vi "Motors Find Datums.vi"(1 "Creep Speed 4":dbl, 2 "Creep Speed 3":dbl, 4 "error in":errorcluster, 5 "Creep Speed 2":dbl, 6 "Creep Speed":dbl, 7 "VISA in":refnum<visa-resource-name>) -> (0 "error out":errorcluster, 3 "VISA out":refnum<visa-resource-name>)   [LabVIEW 2018]
panel:
  out "read buffer":string
  in  "Wait time Theta (s)":i32=1200
  in  "Wait time X (s)":i32=1200
  in  "Wait time Z (s)":i32=1200
  in  "Wait time Y (s)":i32=1200
  out "SV 4":string
  out "DM 4":string
  out "HD 4":string
  out "SV 2":string
  out "HD 1":string
  out "SV 3":string
  out "DM 3":string
  out "HD 3":string
  out "DM 1":string
  out "SV 1":string
  out "HD 2":string
  out "DM 2":string
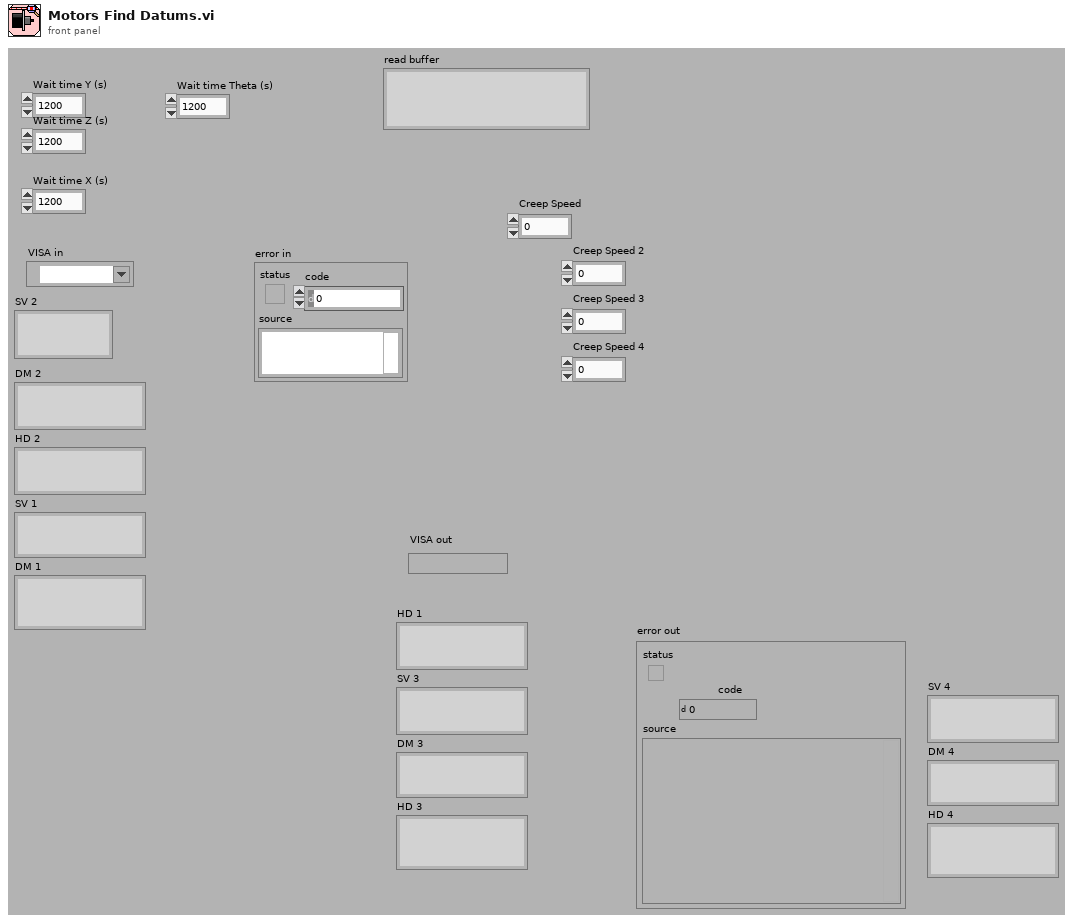
[diagram p1: front panel]
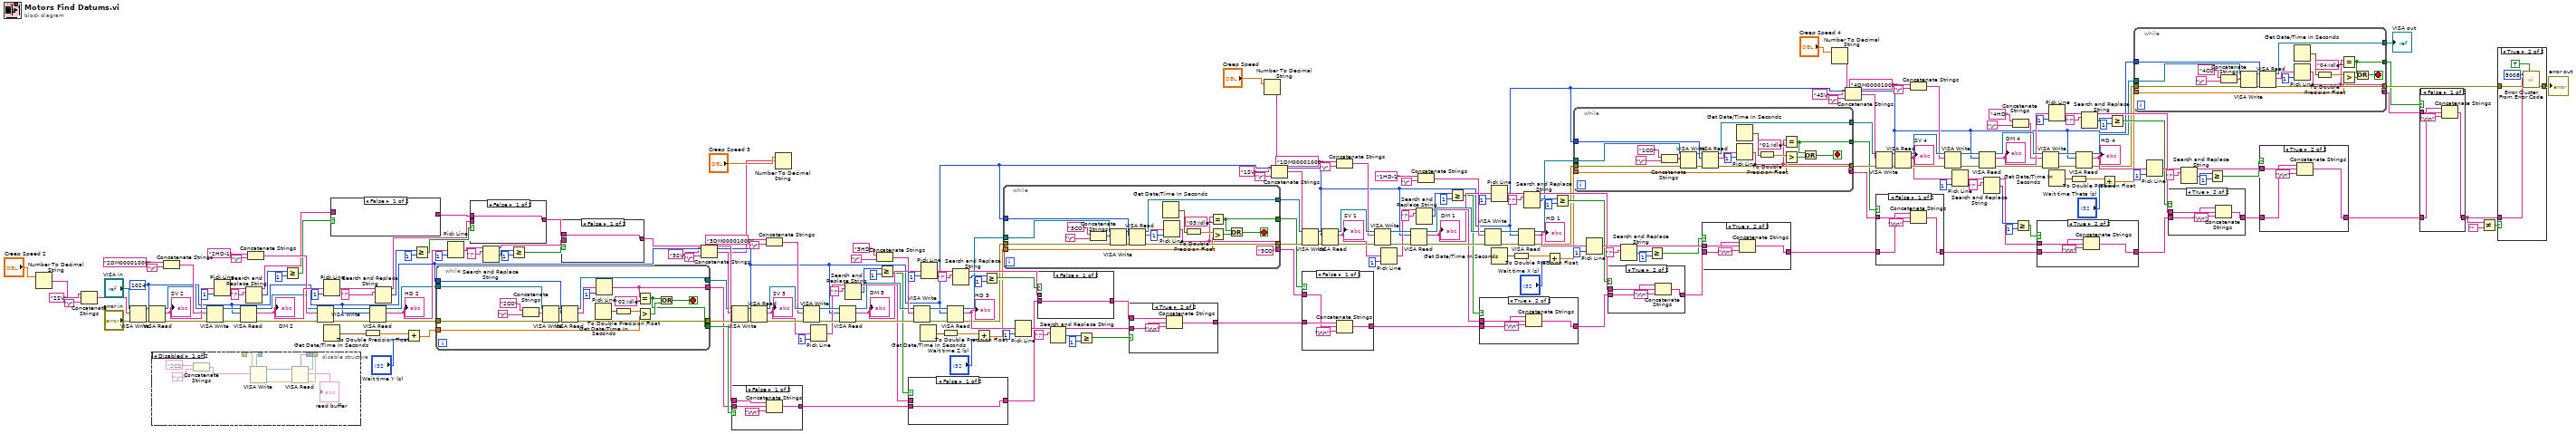
[diagram p0: block diagram]
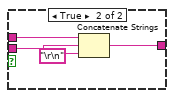
[diagram p8: hidden frame]
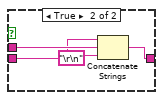
[diagram p13: hidden frame]
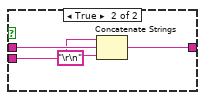
[diagram p14: hidden frame]
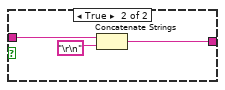
[diagram p18: hidden frame]
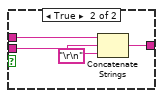
[diagram p19: hidden frame]
diagram:
  w15 = u32 1024 ("byte count")
  n1 = Number To Decimal String(number="Creep Speed 2") -> (decimal integer string=w10:string)  [unwired: 1 in]
  n2 = Concatenate Strings("2SV" ("write buffer"), w10, "\r") -> (w180:string)
  n3 = VISA Write(VISA resource name="VISA in", write buffer=w180, error in (no error)="error in") -> (VISA resource name out=w193:refnum<visa-resource-name>, error out=w192:errorcluster)  [unwired: 1 out]
  n4 = VISA Read(VISA resource name=w193, byte count=w15, error in (no error)=w192) -> (VISA resource name out=w190:refnum<visa-resource-name>, read buffer=w181:string, error out=w188:errorcluster)  [unwired: 1 out]
  "SV 2" <- w181
  n5 = disable-structure shown="Disabled" {
    disable-tunnel: _ -> [w251 _]
    disable-tunnel: _ -> [w250 _]
    disable-tunnel: _ -> [w249 _]
    disable-tunnel: [w248 _] -> _
    disable-tunnel: [w247 _] -> _
    frame Disabled {
      n6 = Concatenate Strings("2CD" ("string"), "\r") -> (w245:string)
      n7 = VISA Write(VISA resource name=w250, write buffer=w245, error in (no error)=w249) -> (VISA resource name out=w253:refnum<visa-resource-name>, error out=w252:errorcluster)  [unwired: 1 out]
      n8 = VISA Read(VISA resource name=w253, byte count=w251, error in (no error)=w252) -> (VISA resource name out=w248:refnum<visa-resource-name>, read buffer=→"read buffer":string, error out=w247:errorcluster)  [unwired: 1 out]
    }
    frame Enabled {
    }
  }
  n9 = Concatenate Strings("2DM00001000" ("Initial command 1"), "\r") -> (w204:string)
  n10 = VISA Write(VISA resource name=w190, write buffer=w204, error in (no error)=w188) -> (VISA resource name out=w239:refnum<visa-resource-name>, error out=w240:errorcluster)  [unwired: 1 out]
  n11 = Pick Line(multi-line string=w181, line index=1) -> (output string=w183:string)  [unwired: 1 in]
  n12 = VISA Read(VISA resource name=w239, byte count=w15, error in (no error)=w240) -> (VISA resource name out=w14:refnum<visa-resource-name>, read buffer=w203:string, error out=w13:errorcluster)  [unwired: 1 out]
  "DM 2" <- w203
  n13 = Search and Replace String(input string=w183, search string="!") -> (result string=w185:string, number of replacements=w186:i32)  [unwired: 6 in, 2 out]
  n14 = Concatenate Strings("2HD-1" ("Initial command 1"), "\r") -> (w194:string)
  n15 = Greater Or Equal?(x=w186, y=1) -> (x >= y?=w68:bool)
  n16 = VISA Write(VISA resource name=w14, write buffer=w194, error in (no error)=w13) -> (VISA resource name out=w238:refnum<visa-resource-name>, error out=w237:errorcluster)  [unwired: 1 out]
  n17 = Get Date/Time In Seconds() -> (seconds since 1Jan1904=w63:timestamp)
  n18 = Pick Line(multi-line string=w203, line index=1) -> (output string=w201:string)  [unwired: 1 in]
  n19 = case shown="False" w68 {
    tunnel: w185 -> [_ w255]
    tunnel: [_ w254] -> w86
    frame False {
    }
    frame True {
      n20 = Concatenate Strings(w255, "\r\n") -> (w254:string)
    }
  }
  n21 = To Double Precision Float(number=w63) -> (double precision float=w62:dbl)
  n22 = VISA Read(VISA resource name=w238, byte count=w15, error in (no error)=w237) -> (VISA resource name out=w64:refnum<visa-resource-name>, read buffer=w87:string, error out=w65:errorcluster)  [unwired: 1 out]
  "HD 2" <- w87
  n23 = Search and Replace String(input string=w201, search string="!") -> (result string=w199:string, number of replacements=w198:i32)  [unwired: 6 in, 2 out]
  n24 = Add(x=w62, y="Wait time Y (s)") -> (x+y=w61:dbl)
  n25 = Greater Or Equal?(x=w198, y=1) -> (x >= y?=w69:bool)
  n26 = while {
    tunnel: w65 -> [w276]
    tunnel: w64 -> [w275]
    tunnel: w15 -> [w261]
    tunnel: [w262] -> w57
    tunnel: [w263] -> w56
    tunnel: w61 -> [w272]
    tunnel: [w268] -> w37
    tunnel: [w266] -> w36
    stop <- w269 stop-if-true
    n27 = Concatenate Strings("2CO" ("write buffer"), "\r") -> (w258:string)
    n28 = VISA Write(VISA resource name=w275, write buffer=w258, error in (no error)=w276) -> (VISA resource name out=w265:refnum<visa-resource-name>, error out=w264:errorcluster)  [unwired: 1 out]
    n29 = VISA Read(VISA resource name=w265, byte count=w261, error in (no error)=w264) -> (VISA resource name out=w262:refnum<visa-resource-name>, read buffer=w260:string, error out=w263:errorcluster)  [unwired: 1 out]
    n30 = Get Date/Time In Seconds() -> (seconds since 1Jan1904=w273:timestamp)
    n31 = Pick Line(multi-line string=w260, line index=1) -> (output string=w266:string)  [unwired: 1 in]
    n32 = To Double Precision Float(number=w273) -> (double precision float=w271:dbl)
    n33 = Equal?(x=w266, y="02:Idle") -> (x = y?=w268:bool)
    n34 = Greater?(x=w271, y=w272) -> (0:w270:bool)
    n35 = Or(x=w268, y=w270) -> (x .or. y?=w269:bool)
  }
  n36 = Pick Line(multi-line string=w87, line index=1) -> (output string=w93:string)  [unwired: 1 in]
  n37 = case shown="False" w69 {
    tunnel: w199 -> [_ w280]
    tunnel: w86 -> [w277 w281]
    tunnel: [w277 w278] -> w85
    frame False {
    }
    frame True {
      n38 = Concatenate Strings(w281, w280, "\r\n") -> (w278:string)
    }
  }
  n39 = Search and Replace String(input string=w93, search string="!") -> (result string=w91:string, number of replacements=w90:i32)  [unwired: 6 in, 2 out]
  n40 = Greater Or Equal?(x=w90, y=1) -> (x >= y?=w67:bool)
  n41 = case shown="False" w67 {
    tunnel: w91 -> [_ w284]
    tunnel: w85 -> [w282 w285]
    tunnel: [w282 w283] -> w35
    frame False {
    }
    frame True {
      n42 = Concatenate Strings(w285, w284, "\r\n") -> (w283:string)
    }
  }
  n43 = case shown="False" w37 {
    tunnel: w36 -> [w288 _]
    tunnel: w35 -> [w289 w291]
    tunnel: [w287 w291] -> w30
    frame False {
      n44 = Concatenate Strings(w289, w288, "\r\n") -> (w287:string)
    }
    frame True {
    }
  }
  n45 = Concatenate Strings("3DM00001000" ("Initial command 3"), "\r") -> (w219:string)
  n46 = Number To Decimal String(number="Creep Speed 3") -> (decimal integer string=w7:string)  [unwired: 1 in]
  n47 = Concatenate Strings("3SV" ("Initial command 2"), w7, "\r") -> (w216:string)
  n48 = VISA Write(VISA resource name=w57, write buffer=w216, error in (no error)=w56) -> (VISA resource name out=w213:refnum<visa-resource-name>, error out=w214:errorcluster)  [unwired: 1 out]
  n49 = VISA Read(VISA resource name=w213, byte count=w15, error in (no error)=w214) -> (VISA resource name out=w221:refnum<visa-resource-name>, read buffer=w147:string, error out=w220:errorcluster)  [unwired: 1 out]
  "SV 3" <- w147
  n50 = VISA Write(VISA resource name=w221, write buffer=w219, error in (no error)=w220) -> (VISA resource name out=w223:refnum<visa-resource-name>, error out=w222:errorcluster)  [unwired: 1 out]
  n51 = Pick Line(multi-line string=w147, line index=1) -> (output string=w152:string)  [unwired: 1 in]
  n52 = VISA Read(VISA resource name=w223, byte count=w15, error in (no error)=w222) -> (VISA resource name out=w224:refnum<visa-resource-name>, read buffer=w140:string, error out=w225:errorcluster)  [unwired: 1 out]
  "DM 3" <- w140
  n53 = Search and Replace String(input string=w152, search string="!") -> (result string=w150:string, number of replacements=w149:i32)  [unwired: 6 in, 2 out]
  n54 = Concatenate Strings("3HD" ("Initial command 4"), "\r") -> (w229:string)
  n55 = Greater Or Equal?(x=w149, y=1) -> (x >= y?=w73:bool)
  n56 = case shown="False" w73 {
    tunnel: w150 -> [_ w295]
    tunnel: [w292 w294] -> w82
    tunnel: w30 -> [w292 w293]
    frame False {
    }
    frame True {
      n57 = Concatenate Strings(w293, w295, "\r\n") -> (w294:string)
    }
  }
  n58 = VISA Write(VISA resource name=w224, write buffer=w229, error in (no error)=w225) -> (VISA resource name out=w227:refnum<visa-resource-name>, error out=w226:errorcluster)  [unwired: 1 out]
  n59 = Get Date/Time In Seconds() -> (seconds since 1Jan1904=w58:timestamp)
  n60 = Pick Line(multi-line string=w140, line index=1) -> (output string=w142:string)  [unwired: 1 in]
  n61 = To Double Precision Float(number=w58) -> (double precision float=w59:dbl)
  n62 = VISA Read(VISA resource name=w227, byte count=w15, error in (no error)=w226) -> (VISA resource name out=w55:refnum<visa-resource-name>, read buffer=w133:string, error out=w54:errorcluster)  [unwired: 1 out]
  "HD 3" <- w133
  n63 = Search and Replace String(input string=w142, search string="!") -> (result string=w144:string, number of replacements=w145:i32)  [unwired: 6 in, 2 out]
  n64 = Add(x=w59, y="Wait time Z (s)") -> (x+y=w60:dbl)
  n65 = Greater Or Equal?(x=w145, y=1) -> (x >= y?=w74:bool)
  n66 = while {
    tunnel: w54 -> [w316]
    tunnel: w55 -> [w303]
    tunnel: w15 -> [w315]
    tunnel: [w309] -> w53
    tunnel: [w308] -> w52
    tunnel: w60 -> [w306]
    tunnel: [w301] -> w34
    tunnel: [w300] -> w33
    stop <- w304 stop-if-true
    (unwired) "3CO" ("write buffer")
    n67 = Concatenate Strings("3CO" ("write buffer"), "\r") -> (w297:string)
    n68 = VISA Write(VISA resource name=w303, write buffer=w297, error in (no error)=w316) -> (VISA resource name out=w314:refnum<visa-resource-name>, error out=w313:errorcluster)  [unwired: 1 out]
    n69 = VISA Read(VISA resource name=w314, byte count=w315, error in (no error)=w313) -> (VISA resource name out=w309:refnum<visa-resource-name>, read buffer=w311:string, error out=w308:errorcluster)  [unwired: 1 out]
    n70 = Get Date/Time In Seconds() -> (seconds since 1Jan1904=w307:timestamp)
    n71 = Pick Line(multi-line string=w311, line index=1) -> (output string=w300:string)  [unwired: 1 in]
    n72 = To Double Precision Float(number=w307) -> (double precision float=w302:dbl)
    n73 = Equal?(x=w300, y="03:Idle") -> (x = y?=w301:bool)
    n74 = Greater?(x=w302, y=w306) -> (0:w305:bool)
    n75 = Or(x=w301, y=w305) -> (x .or. y?=w304:bool)
  }
  n76 = Pick Line(multi-line string=w133, line index=1) -> (output string=w138:string)  [unwired: 1 in]
  n77 = case shown="False" w74 {
    tunnel: w144 -> [_ w320]
    tunnel: [w317 w319] -> w81
    tunnel: w82 -> [w317 w318]
    frame False {
    }
    frame True {
      n78 = Concatenate Strings(w318, w320, "\r\n") -> (w319:string)
    }
  }
  n79 = Search and Replace String(input string=w138, search string="!") -> (result string=w136:string, number of replacements=w135:i32)  [unwired: 6 in, 2 out]
  n80 = Greater Or Equal?(x=w135, y=1) -> (x >= y?=w75:bool)
  n81 = case shown="True" w75 {
    tunnel: w136 -> [_ w325]
    tunnel: w81 -> [w322 w324]
    tunnel: [w322 w323] -> w32
    frame False {
    }
    frame True {
      n82 = Concatenate Strings(w324, w325, "\r\n") -> (w323:string)
    }
  }
  n83 = Number To Decimal String(number="Creep Speed") -> (decimal integer string=w4:string)  [unwired: 1 in]
  n84 = Concatenate Strings("1SV" ("write buffer"), w4, "\r") -> (w177:string)
  n85 = VISA Write(VISA resource name=w53, write buffer=w177, error in (no error)=w52) -> (VISA resource name out=w235:refnum<visa-resource-name>, error out=w236:errorcluster)  [unwired: 1 out]
  n86 = case shown="False" w34 {
    tunnel: w33 -> [w328 _]
    tunnel: w32 -> [w329 w331]
    tunnel: [w327 w331] -> w31
    frame False {
      n87 = Concatenate Strings(w329, w328, "\r\n") -> (w327:string)
    }
    frame True {
    }
  }
  n88 = VISA Read(VISA resource name=w235, byte count=w15, error in (no error)=w236) -> (VISA resource name out=w234:refnum<visa-resource-name>, read buffer=w170:string, error out=w233:errorcluster)  [unwired: 1 out]
  "SV 1" <- w170
  n89 = Concatenate Strings("1DM00001000" ("Initial command 1"), "\r") -> (w169:string)
  n90 = VISA Write(VISA resource name=w234, write buffer=w169, error in (no error)=w233) -> (VISA resource name out=w231:refnum<visa-resource-name>, error out=w232:errorcluster)  [unwired: 1 out]
  n91 = Pick Line(multi-line string=w170, line index=1) -> (output string=w172:string)  [unwired: 1 in]
  n92 = VISA Read(VISA resource name=w231, byte count=w15, error in (no error)=w232) -> (VISA resource name out=w208:refnum<visa-resource-name>, read buffer=w162:string, error out=w207:errorcluster)  [unwired: 1 out]
  "DM 1" <- w162
  n93 = Search and Replace String(input string=w172, search string="!") -> (result string=w174:string, number of replacements=w175:i32)  [unwired: 6 in, 2 out]
  n94 = Concatenate Strings("1HD-1" ("Initial command 1"), "\r") -> (w210:string)
  n95 = Greater Or Equal?(x=w175, y=1) -> (x >= y?=w70:bool)
  n96 = case shown="True" w70 {
    tunnel: w174 -> [_ w335]
    tunnel: [w332 w334] -> w84
    tunnel: w31 -> [w332 w333]
    frame False {
    }
    frame True {
      n97 = Concatenate Strings(w333, w335, "\r\n") -> (w334:string)
    }
  }
  n98 = VISA Write(VISA resource name=w208, write buffer=w210, error in (no error)=w207) -> (VISA resource name out=w212:refnum<visa-resource-name>, error out=w211:errorcluster)  [unwired: 1 out]
  n99 = Get Date/Time In Seconds() -> (seconds since 1Jan1904=w51:timestamp)
  n100 = Pick Line(multi-line string=w162, line index=1) -> (output string=w167:string)  [unwired: 1 in]
  n101 = To Double Precision Float(number=w51) -> (double precision float=w50:dbl)
  n102 = VISA Read(VISA resource name=w212, byte count=w15, error in (no error)=w211) -> (VISA resource name out=w48:refnum<visa-resource-name>, read buffer=w154:string, error out=w47:errorcluster)  [unwired: 1 out]
  "HD 1" <- w154
  n103 = Search and Replace String(input string=w167, search string="!") -> (result string=w165:string, number of replacements=w164:i32)  [unwired: 6 in, 2 out]
  n104 = Add(x=w50, y="Wait time X (s)") -> (x+y=w49:dbl)
  n105 = Greater Or Equal?(x=w164, y=1) -> (x >= y?=w71:bool)
  n106 = while {
    tunnel: w47 -> [w356]
    tunnel: w48 -> [w342]
    tunnel: w15 -> [w355]
    tunnel: [w349] -> w46
    tunnel: [w348] -> w45
    tunnel: w49 -> [w346]
    tunnel: [w341] -> w29
    tunnel: [w340] -> w27
    stop <- w343 stop-if-true
    n107 = Concatenate Strings("1CO" ("write buffer"), "\r") -> (w337:string)
    n108 = VISA Write(VISA resource name=w342, write buffer=w337, error in (no error)=w356) -> (VISA resource name out=w354:refnum<visa-resource-name>, error out=w353:errorcluster)  [unwired: 1 out]
    n109 = VISA Read(VISA resource name=w354, byte count=w355, error in (no error)=w353) -> (VISA resource name out=w349:refnum<visa-resource-name>, read buffer=w351:string, error out=w348:errorcluster)  [unwired: 1 out]
    n110 = Get Date/Time In Seconds() -> (seconds since 1Jan1904=w347:timestamp)
    n111 = Pick Line(multi-line string=w351, line index=1) -> (output string=w341:string)  [unwired: 1 in]
    n112 = To Double Precision Float(number=w347) -> (double precision float=w345:dbl)
    n113 = Equal?(x=w341, y="01:Idle") -> (x = y?=w340:bool)
    n114 = Greater?(x=w345, y=w346) -> (0:w344:bool)
    n115 = Or(x=w340, y=w344) -> (x .or. y?=w343:bool)
  }
  n116 = Pick Line(multi-line string=w154, line index=1) -> (output string=w156:string)  [unwired: 1 in]
  n117 = case shown="True" w71 {
    tunnel: w165 -> [_ w360]
    tunnel: [w357 w359] -> w83
    tunnel: w84 -> [w357 w358]
    frame False {
    }
    frame True {
      n118 = Concatenate Strings(w358, w360, "\r\n") -> (w359:string)
    }
  }
  n119 = Search and Replace String(input string=w156, search string="!") -> (result string=w158:string, number of replacements=w159:i32)  [unwired: 6 in, 2 out]
  n120 = Greater Or Equal?(x=w159, y=1) -> (x >= y?=w72:bool)
  n121 = case shown="True" w72 {
    tunnel: w158 -> [_ w365]
    tunnel: [w362 w364] -> w28
    tunnel: w83 -> [w362 w363]
    frame False {
    }
    frame True {
      n122 = Concatenate Strings(w363, w365, "\r\n") -> (w364:string)
    }
  }
  n123 = Number To Decimal String(number="Creep Speed 4") -> (decimal integer string=w1:string)  [unwired: 1 in]
  n124 = Concatenate Strings("4SV" ("Initial command 2"), w1, "\r") -> (w121:string)
  n125 = VISA Write(VISA resource name=w46, write buffer=w121, error in (no error)=w45) -> (VISA resource name out=w132:refnum<visa-resource-name>, error out=w131:errorcluster)  [unwired: 1 out]
  n126 = case shown="False" w27 {
    tunnel: w29 -> [w368 _]
    tunnel: w28 -> [w369 w371]
    tunnel: [w367 w371] -> w26
    frame False {
      n127 = Concatenate Strings(w369, w368, "\r\n") -> (w367:string)
    }
    frame True {
    }
  }
  n128 = VISA Read(VISA resource name=w132, byte count=w15, error in (no error)=w131) -> (VISA resource name out=w129:refnum<visa-resource-name>, read buffer=w114:string, error out=w130:errorcluster)  [unwired: 1 out]
  "SV 4" <- w114
  n129 = Concatenate Strings("4DM00001000" ("Initial command 3"), "\r") -> (w111:string)
  n130 = VISA Write(VISA resource name=w129, write buffer=w111, error in (no error)=w130) -> (VISA resource name out=w127:refnum<visa-resource-name>, error out=w128:errorcluster)  [unwired: 1 out]
  n131 = Pick Line(multi-line string=w114, line index=1) -> (output string=w116:string)  [unwired: 1 in]
  n132 = VISA Read(VISA resource name=w127, byte count=w15, error in (no error)=w128) -> (VISA resource name out=w126:refnum<visa-resource-name>, read buffer=w104:string, error out=w125:errorcluster)  [unwired: 1 out]
  "DM 4" <- w104
  n133 = Search and Replace String(input string=w116, search string="!") -> (result string=w118:string, number of replacements=w119:i32)  [unwired: 6 in, 2 out]
  n134 = Concatenate Strings("4HD" ("Initial command 4"), "\r") -> (w101:string)
  n135 = Greater Or Equal?(x=w119, y=1) -> (x >= y?=w76:bool)
  n136 = case shown="True" w76 {
    tunnel: w118 -> [_ w375]
    tunnel: [w372 w374] -> w80
    tunnel: w26 -> [w372 w373]
    frame False {
    }
    frame True {
      n137 = Concatenate Strings(w373, w375, "\r\n") -> (w374:string)
    }
  }
  n138 = VISA Write(VISA resource name=w126, write buffer=w101, error in (no error)=w125) -> (VISA resource name out=w123:refnum<visa-resource-name>, error out=w124:errorcluster)  [unwired: 1 out]
  n139 = Get Date/Time In Seconds() -> (seconds since 1Jan1904=w42:timestamp)
  n140 = Pick Line(multi-line string=w104, line index=1) -> (output string=w109:string)  [unwired: 1 in]
  n141 = To Double Precision Float(number=w42) -> (double precision float=w43:dbl)
  n142 = VISA Read(VISA resource name=w123, byte count=w15, error in (no error)=w124) -> (VISA resource name out=w41:refnum<visa-resource-name>, read buffer=w94:string, error out=w40:errorcluster)  [unwired: 1 out]
  "HD 4" <- w94
  n143 = Search and Replace String(input string=w109, search string="!") -> (result string=w107:string, number of replacements=w106:i32)  [unwired: 6 in, 2 out]
  n144 = Add(x=w43, y="Wait time Theta (s)") -> (x+y=w44:dbl)
  n145 = Greater Or Equal?(x=w106, y=1) -> (x >= y?=w77:bool)
  n146 = while {
    tunnel: w40 -> [w396]
    tunnel: w41 -> [w384]
    tunnel: [w390] -> w39
    tunnel: [w389] -> w38
    tunnel: w44 -> [w387]
    tunnel: w15 -> [w383]
    tunnel: [w381] -> w25
    tunnel: [w380] -> w24
    stop <- w385 stop-if-true
    n147 = Concatenate Strings("4CO" ("write buffer"), "\r") -> (w377:string)
    n148 = VISA Write(VISA resource name=w384, write buffer=w377, error in (no error)=w396) -> (VISA resource name out=w395:refnum<visa-resource-name>, error out=w394:errorcluster)  [unwired: 1 out]
    n149 = VISA Read(VISA resource name=w395, byte count=w383, error in (no error)=w394) -> (VISA resource name out=w390:refnum<visa-resource-name>, read buffer=w392:string, error out=w389:errorcluster)  [unwired: 1 out]
    n150 = Get Date/Time In Seconds() -> (seconds since 1Jan1904=w388:timestamp)
    n151 = Pick Line(multi-line string=w392, line index=1) -> (output string=w381:string)  [unwired: 1 in]
    n152 = To Double Precision Float(number=w388) -> (double precision float=w382:dbl)
    n153 = Equal?(x=w381, y="04:Idle") -> (x = y?=w380:bool)
    n154 = Greater?(x=w382, y=w387) -> (0:w386:bool)
    n155 = Or(x=w380, y=w386) -> (x .or. y?=w385:bool)
  }
  "VISA out" <- w39
  n156 = Pick Line(multi-line string=w94, line index=1) -> (output string=w96:string)  [unwired: 1 in]
  n157 = case shown="True" w77 {
    tunnel: w107 -> [_ w400]
    tunnel: [w397 w398] -> w79
    tunnel: w80 -> [w397 w399]
    frame False {
    }
    frame True {
      n158 = Concatenate Strings(w399, w400, "\r\n") -> (w398:string)
    }
  }
  n159 = Search and Replace String(input string=w96, search string="!") -> (result string=w98:string, number of replacements=w99:i32)  [unwired: 6 in, 2 out]
  n160 = Greater Or Equal?(x=w99, y=1) -> (x >= y?=w78:bool)
  n161 = case shown="True" w78 {
    tunnel: w98 -> [_ w405]
    tunnel: w79 -> [w402 w404]
    tunnel: [w402 w403] -> w23
    frame False {
    }
    frame True {
      n162 = Concatenate Strings(w404, w405, "\r\n") -> (w403:string)
    }
  }
  n163 = case shown="False" w24 {
    tunnel: w25 -> [w408 _]
    tunnel: w23 -> [w409 w411]
    tunnel: [w407 w411] -> w22
    frame False {
      n164 = Concatenate Strings(w409, w408, "\r\n") -> (w407:string)
    }
    frame True {
    }
  }
  n165 = Not Equal?(x=w22, y="") -> (x != y?=w20:bool)
  n166 = case shown="True" w20 {
    tunnel: [w412 w416] -> w66
    tunnel: w38 -> [w412 w417]
    tunnel: w22 -> [_ w413]
    frame False {
    }
    frame True {
      n167 = call <vilib>:"Error Cluster From Error Code.vi"("show call chain? (False)"=TRUE, "error in (no error)"=w417, "error message (\"\")"=w413, "error code (0)"=5008) -> ("error out"=w416:errorcluster)  [unwired: 5 in]
    }
  }
  "error out" <- w66
